vi "SiPM_Data_Analysis.vi"() -> ()   [LabVIEW 2019]
uses:
  <vilib>/Utility/error.llb/DialogType.ctl
  SiPM_Tests_Global_Var.vi
  Data_Analysis_subvis/ESA_Data_Analysis_Global_VIs.vi
  <vilib>/Analysis/NI_AALPro.lvlib
panel:
  out "property names":string[](array[string])
  out "property values":variant[](array[variant])
  out "data":waveform(dbl)[](array[waveform])
  out "Indicator":bool
  in  "Close Session":bool
  in  "Spectrum Calculation":bool=TRUE
  in  "Waveform Nb":u16
  in  "NbSamples":i64=100000 caption="Nb of Samples to Analyze" format="%.0p"
  in  "Refresh":bool
  in  "Load file to display":bool
  in  "Detailed":bool
  in  "Listbox":i32[](listbox) caption="Proton-Neutron_Brd.tdms"
  in  "Tab Control":enum32{"Waveform", "Calibration"}(tab)
  out "SiPM Waveform":waveform(dbl)[](graph)
  in  "X-Scale":bool
  in  "Calibrate":bool
  out "Offset":dbl step=0.001 format="%#_6p"
  out "Gain":dbl step=0.001 format="%#_6p"
  in  "Y2 (keV)":dbl
  in  "Y1 (keV)":dbl
  in  "AutoScale 4":bool
  out "Waveform Graph":dbl[][](graph)
  in  "Lower Cut-Off":dbl=50.0
  in  "Y-Scale 2":bool caption="Y-Scale"
  in  "CH1 Trigger Logic":T1(ring)=enum."Don't Care"
  in  "CH1 Trigger Thr":dbl=0.003 caption="CH1 Trigger Thr (V)" step=0.001 format="%#_6p"
  in  "Y-Scale":bool
  out "Nb of Selected Events":dbl step=0.001 format="%#_6p"
  out "Total Nb of Recorded Events":dbl step=0.001 format="%#_6p"
  in  "CH4 Trigger Logic":T1(ring)
  in  "CH4 Trigger Thr":dbl=0.003 caption="CH4 Trigger Thr (V)" step=0.001 format="%#_6p"
  in  "CH3 Trigger Logic":T1(ring)
  in  "CH3 Trigger":dbl=0.003 caption="CH3 Trigger Thr (V)" step=0.001 format="%#_6p"
  in  "CH2 Trigger Logic":T1(ring)=enum."Don't Care"
  in  "CH2 Trigger Thr":dbl=0.003 caption="CH2 Trigger Thr (V)" step=0.001 format="%#_6p"
  in  "AutoScale 3":bool
  in  "Update Energy":bool
  out "Energy_Spectr":T2(graph) caption="Spectrum"
  in  "Filter \nON?":bool
  in  "Threshold 2":dbl caption="Max_Value (V)" step=0.001 format="%#_6p"
  in  "Threshold":dbl caption="Energy Threshold (V)" step=0.001 format="%#_6p"
  out "Table":string[][](table)
  in  "Bin Min (V)":dbl=-0.0042 step=0.001 format="%#_6p"
  in  "Bin Max (V)":dbl=0.03005 step=0.001 format="%#_6p"
  out "Nb of Channels in Group":i32
  out "group names":string[](array[string])
  out "tdms file out":refnum<k34>
  in  "File contents":string[](tree)
  # "NCSR  DEMOKRITOS\nInstitute of Nuclear and Particle Physics\nDetectors Instrumentation Laboratory"
  # "SiPM Data Analysis"
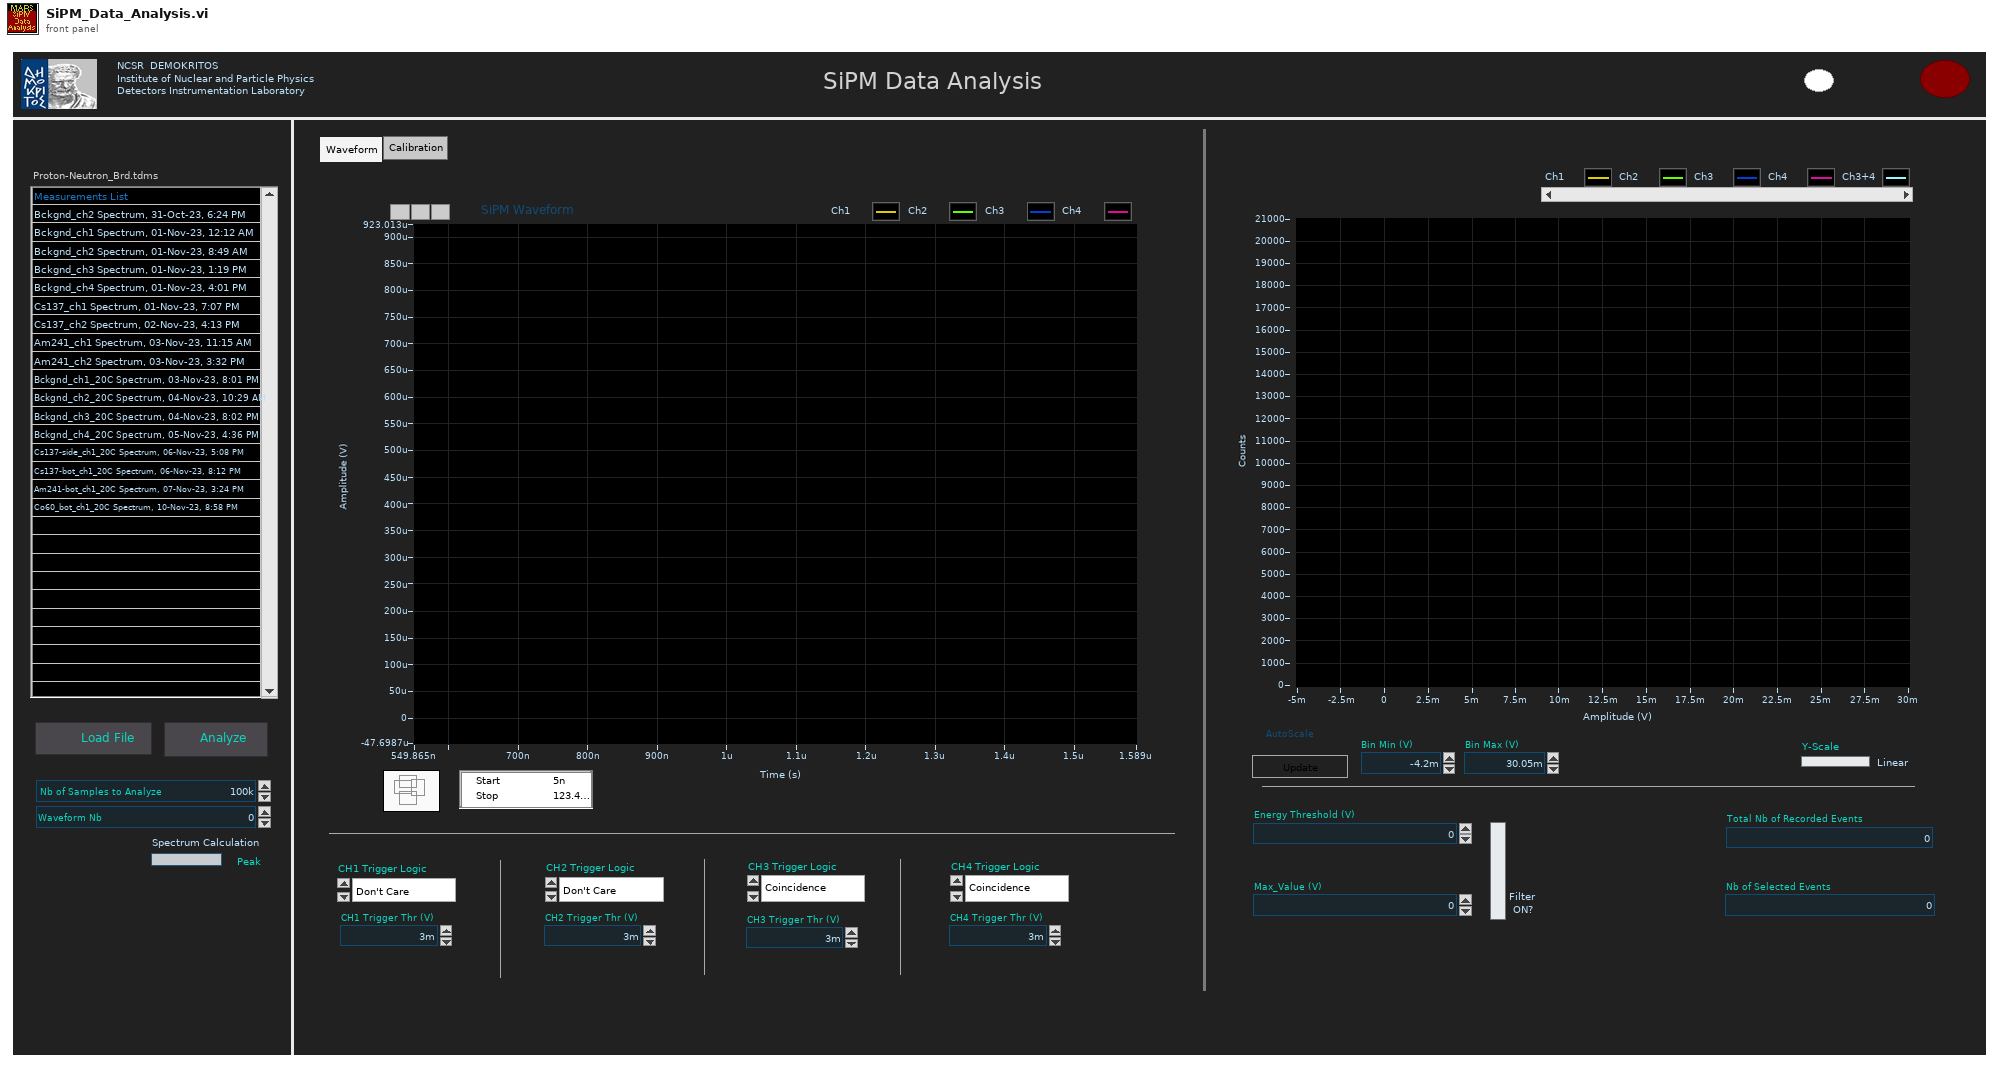
[diagram p1: front panel]
types:
  T1 = enum16{"Coincidence", "Anti-Coincidence", "Don't Care"}
  T2 = cluster{"X Values":dbl[], "Histogram: h(x)":i32[]}[]
  T3 = typedef "DialogType.ctl" = u16
  T4 = enum16{"open", "open or create", "create or replace", "create", "open (read-only)"}
  T5 = cluster{"X Values":dbl[], "Histogram: h(x)":i32[]}
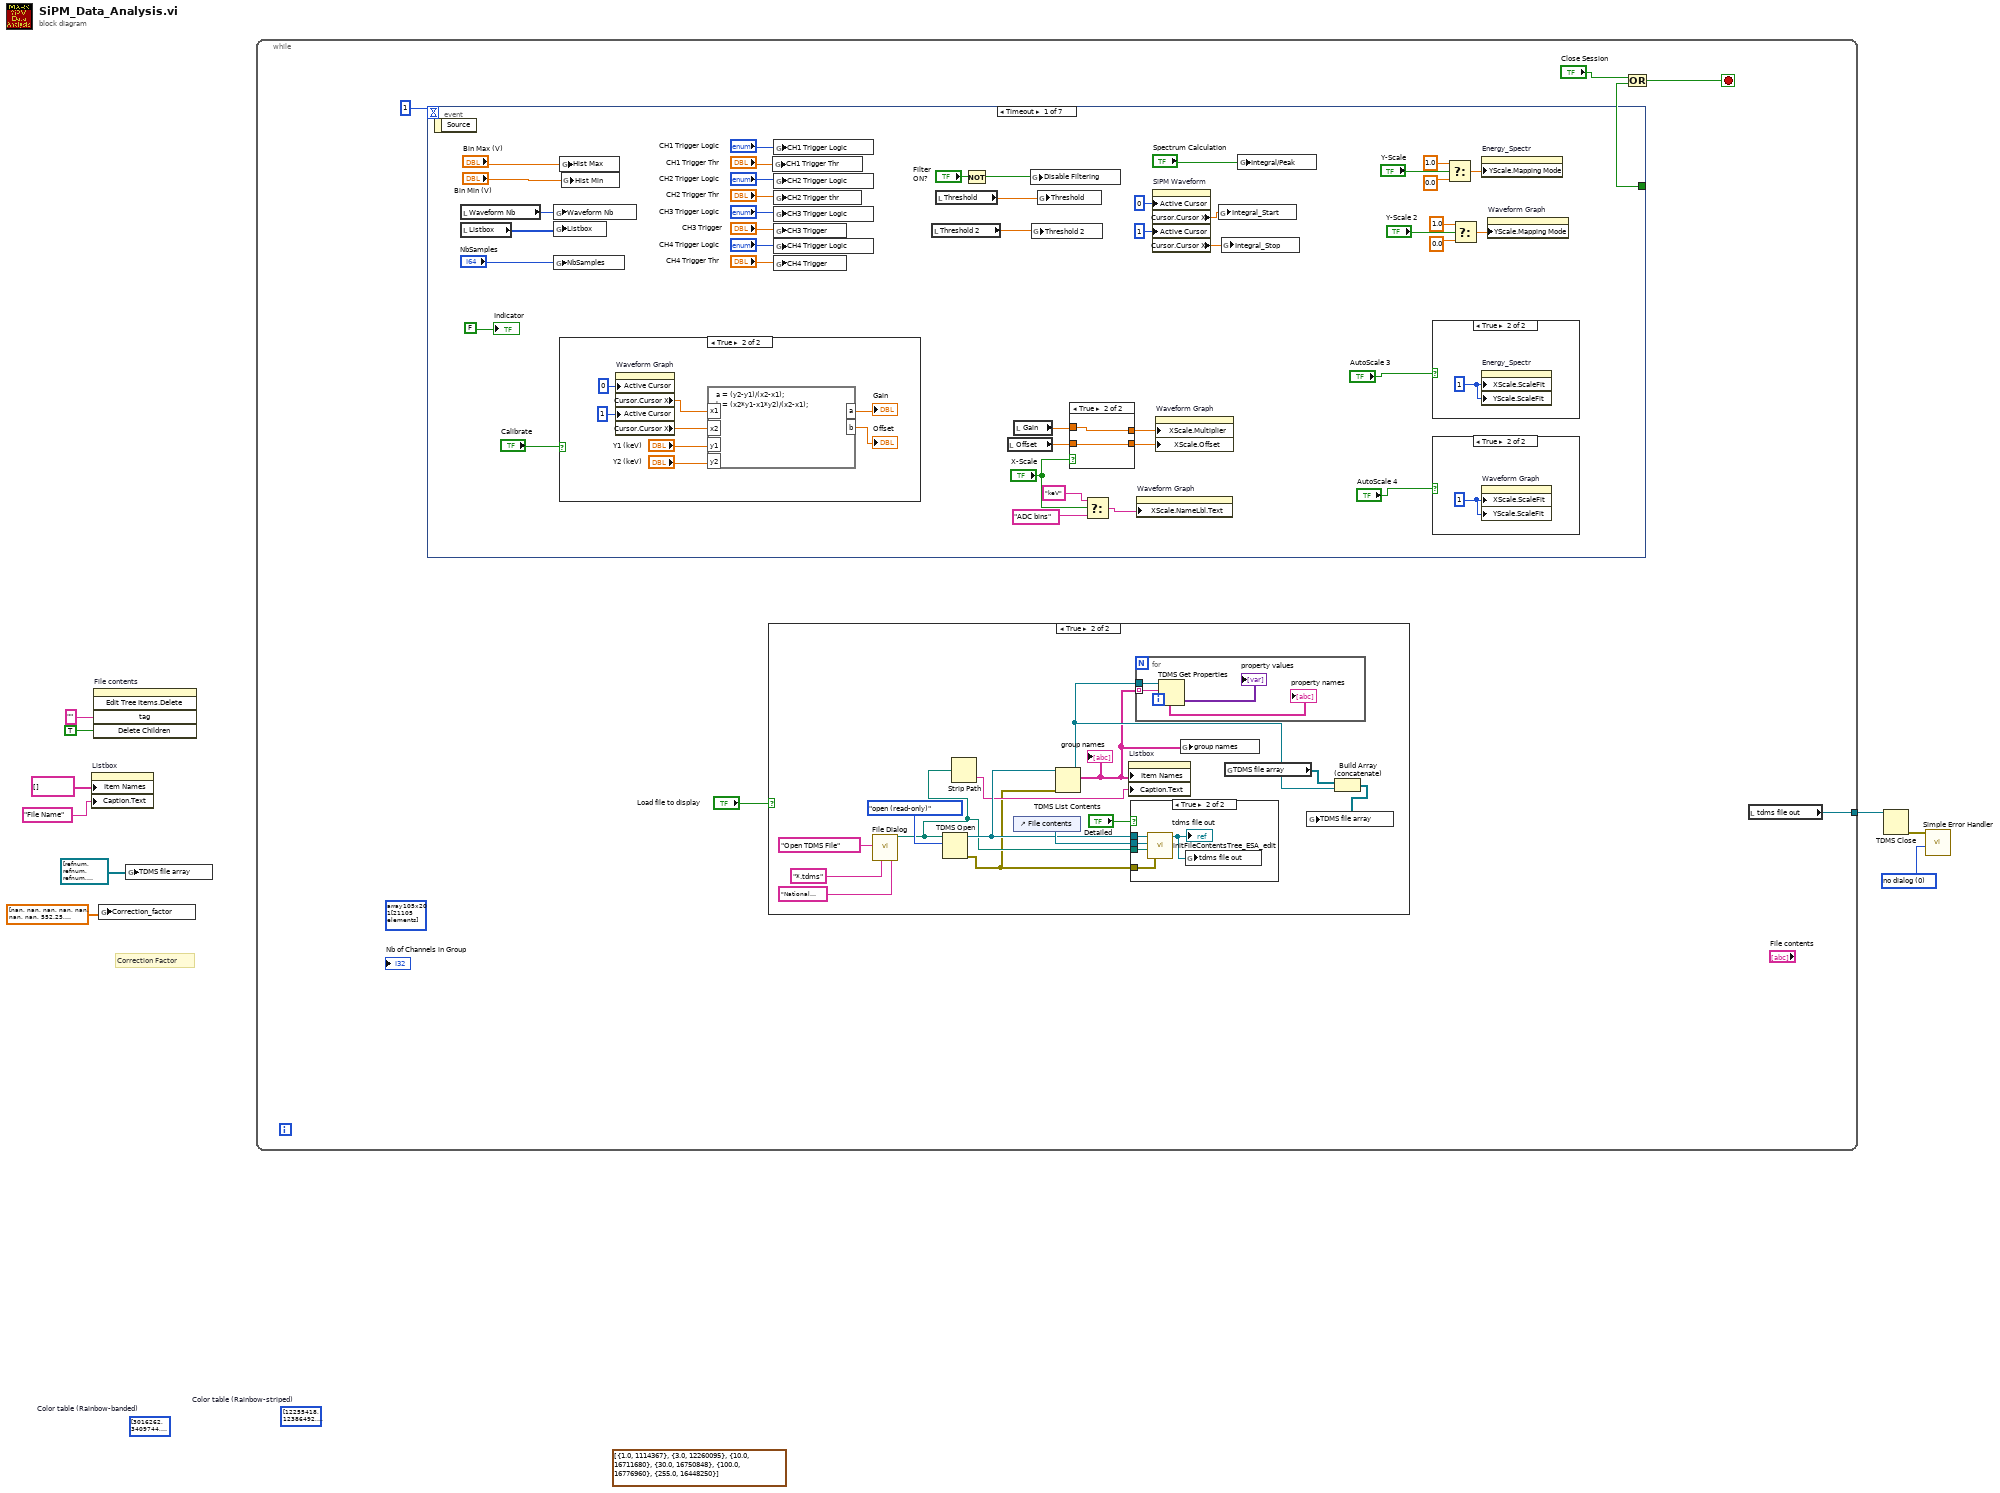
[diagram p0: block diagram]
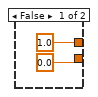
[diagram p2: hidden frame]
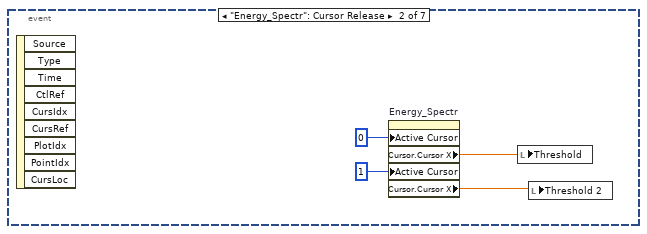
[diagram p6: hidden frame]
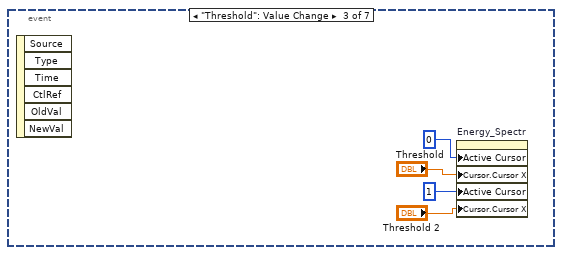
[diagram p7: hidden frame]
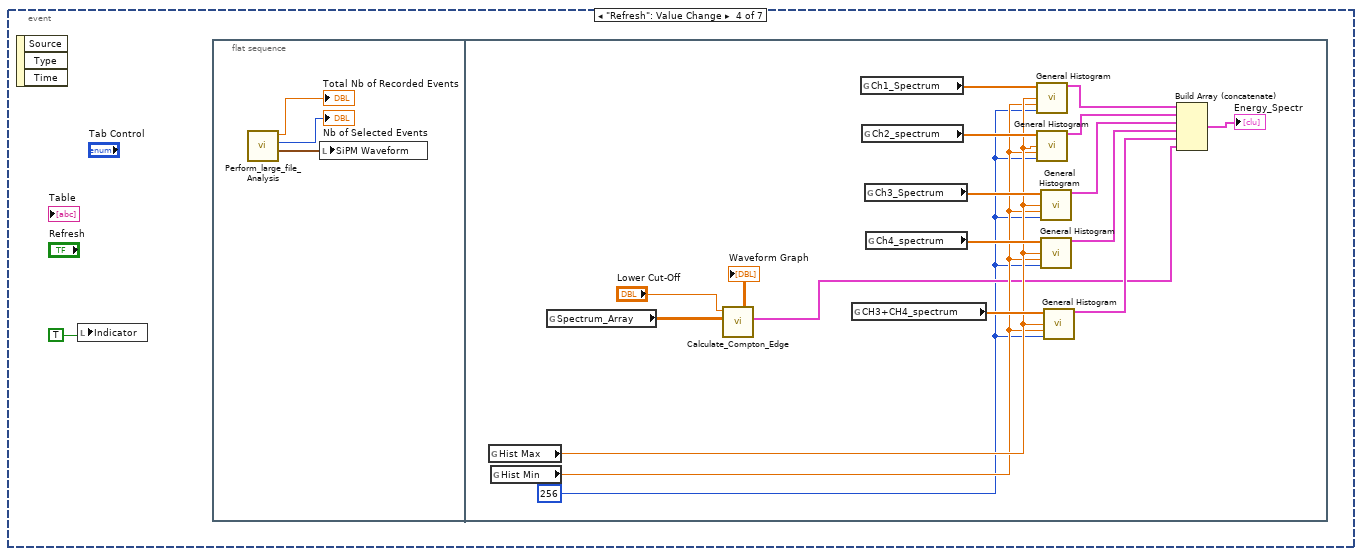
[diagram p8: hidden frame]
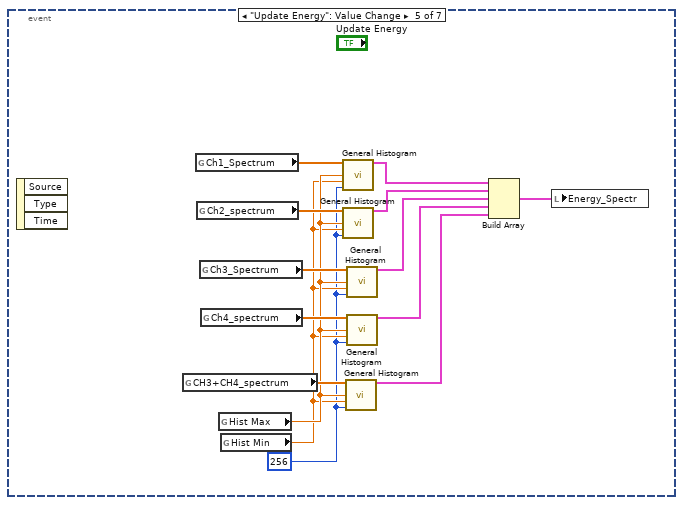
[diagram p9: hidden frame]
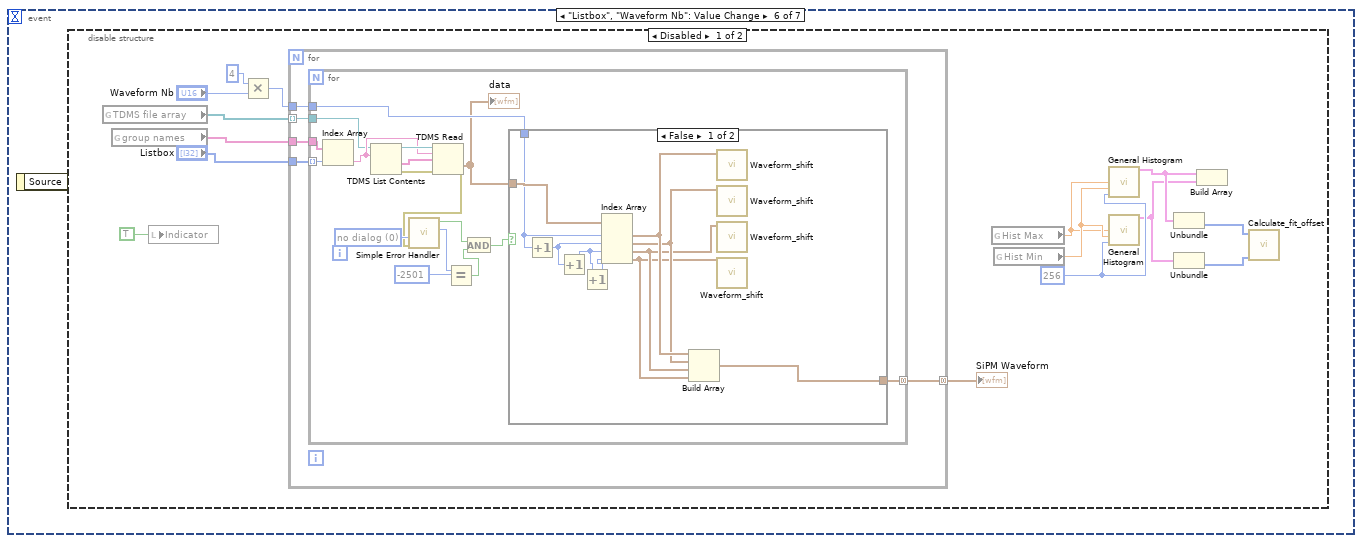
[diagram p10: hidden frame]
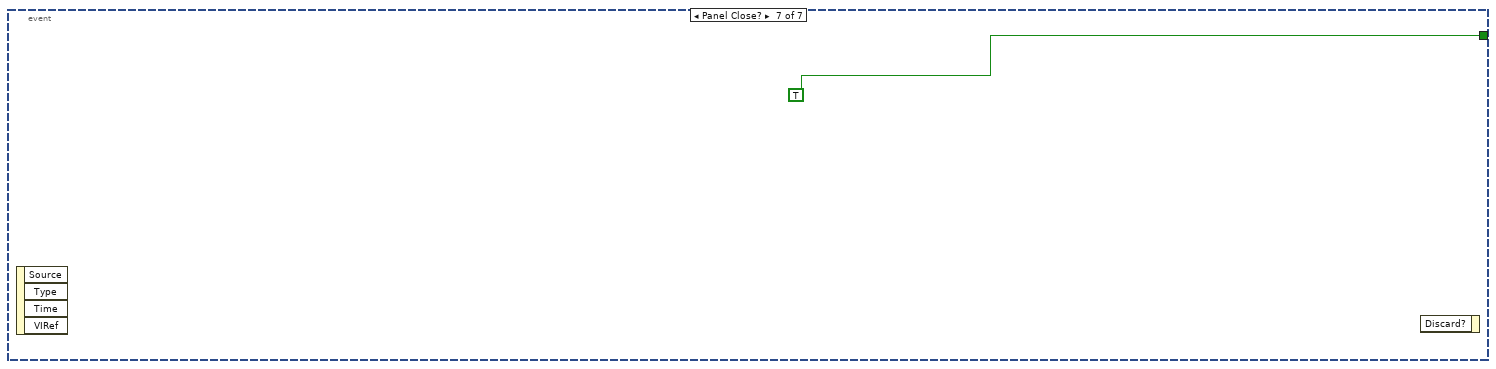
[diagram p13: hidden frame]
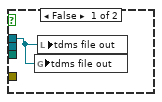
[diagram p15: hidden frame]
diagram:
  w2 = T3 0 items=["no dialog", "OK message", "continue or stop message", "OK message + warnings", "continue/stop + warnings"] ("type of dialog (OK msg:1)")
  (unwired) cluster{dbl, u32}[] [{1.0, 1114367}, {3.0, 12260095}, {10.0, 16711680}, {30.0, 16750848}, {100.0, 16776960}, {255.0, 16448250}] ("Z Scale.Marker Values[]")
  (unwired) u32[] [12255418, 12386492, 12517567, 12320960, 12189888, 12058817, 11927746, 11731139, 11600067, 9175197, 9044125, 11141318, 11010246, 10813639, 10682568, 10551497, 10354890, 10223818, 10092747, 7930019, 7798948, 9633997, 9502926, 9306319, 9175248, 9044176, 8847569, 8716498, 8585427, 6750377, 6619306, 8126677, 7995606, 7798999, 7667927, 7536856, 7340249, 7209178, 7078106, 5505199, 5374128, 6619357, 6488285, 6291678, 6160607, 6029536, 5832929, 5701857, 5570786, 4325557, 4194486, 5112036, 4980965, 4784358, 4653287, 4522215, 4325608, 4194537, 4063466, 3080380, 3014844, 3604716, 3408109, 3277038, 3277038, 3145966, 3014895, 2818288, 2687217, 2556145, 1900738, 1769666, 2097396, 1900789, 1769717, 1638646, 1507575, 1310968, 1179896, 1048825, 721096, 590024, 590075, 393468, 262397, 131326, 255, 1791, 3327, 4863, 5068, 6348, 9471, 11007, 12543, 14079, 15615, 17151, 18687, 20223, 17612, 18636, 25087, 26623, 28159, 29695, 31231, 32767, 34303, 35839, 29900, 31180, 40447, 41983, 43775, 45311, 46847, 48383, 49919, 51455, 42444, 43724, 56063, 57599, 59135, 60671, 62207, 63743, 65535, 65528, 52418, 52413, 65510, 65504, 65498, 65492, 65486, 65480, 65474, 65468, 52369, 52364, 65449, 65443, 65437, 65431, 65425, 65419, 65413, 65407, 52321, 52316, 65389, 65383, 65377, 65371, 65364, 65358, 65352, 65346, 52272, 52267, 65328, 65322, 65316, 65310, 65304, 65298, 65292, 65286, 52224, 314368, 851712, 1244928, 1638144, 2031360, 2424576, 2817792, 3211008, 3604224, 3197952, 3525632, 4783872, 5177088, 5635840, 6029056, 6422272, 6815488, 7208704, 7601920, 6409216, 6736896, 6736896, 8781568, 9174784, 9568000, 9961216, 10354432, 10747648, 11206400, 11599616, 9554944, 9882624, 12779264, 13172480, 13565696, 13958912, 14352128, 14745344, 15138560, 15531776, 12766208, 13093888, 16776960, 16775170, 16773637, 16771847, 16770314, 16768780, 16766991, 16765457, 13411088, 13409810, 16760601, 16758812, 16757278, 16755745, 16753955, 16752422, 16750888, 16749099, 13398052, 13396774, 16744243, 16742704, 16741166, 16739884, 16738345, 16736807, 16735269, 16733730, 13385753, 13384728, 16729371, 16727833, 16726295, 16725012, 16723474, 16721936, 16720397, 16718859, 13373959, 13372677, 16714500, 16712962, 16711680]  # Color table (Rainbow-striped)
  (unwired) u32[] [3016262, 3409744, 4000097, 4721526, 5508493, 6229924, 6820281, 7214025, 7345364, 7279831, 6886611, 6362057, 5640632, 4788132, 4001165, 3214197, 2492769, 2033488, 1640006, 1508930, 1508934, 1640272, 1902945, 2165622, 2428301, 2690980, 2822585, 2888649, 2757844, 2626775, 2299091, 1971145, 1642936, 1249188, 920973, 724086, 592737, 461392, 395846, 396098, 396358, 462928, 595297, 727925, 861069, 994212, 1127608, 1260745, 1328083, 1329111, 1329876, 1264073, 1132217, 999844, 866957, 734070, 600929, 468304, 401734, 401730, 402502, 469584, 603489, 737909, 737909, 872845, 1008036, 1143224, 1277641, 1345747, 1347287, 1347796, 1281225, 1147833, 1013668, 878989, 743798, 609121, 475216, 407878, 407362, 408390, 476496, 611681, 747893, 884877, 1022116, 1158840, 1294793, 1363667, 1365719, 1365202, 1296836, 1161649, 1025178, 888194, 751211, 614742, 479302, 411196, 410168, 411193, 479297, 614732, 750939, 888171, 1025145, 1161350, 1296782, 1364883, 1365906, 1365132, 1296769, 1161588, 1025124, 888147, 751172, 614710, 479276, 411173, 410146, 411170, 479270, 614700, 750900, 888124, 1025091, 1161289, 1296716, 1364813, 1365834, 1365062, 1296703, 1161527, 1025070, 888101, 751133, 614678, 479249, 411149, 410124, 411147, 479244, 614668, 750861, 888078, 1156111, 1488913, 1820947, 2151188, 2414356, 2610196, 2738451, 2668817, 2597903, 2329869, 2061835, 1794313, 1593351, 1459718, 1458694, 1590790, 1921031, 2449673, 3110155, 3902733, 4695055, 5486609, 6211859, 6738708, 7132948, 7197716, 7063827, 6666513, 6136847, 5410061, 4617739, 3957001, 3362823, 2967046, 2900486, 3098118, 3690503, 4546825, 5666059, 6917389, 8233999, 9484305, 10537235, 11326228, 11786004, 11785236, 11785236, 11454739, 10729745, 9675791, 8424717, 7173643, 6054153, 5066759, 4474374, 4342278, 4605190, 5262855, 6380553, 7695883, 9273613, 10785807, 12100625, 13217555, 13874452, 14136340, 13938196, 13214227, 12161553, 10780431, 9267725, 7755531, 6374921, 5257479, 4599814, 4336646, 4599302, 5255943, 6372361, 7685899, 9261837, 10771983, 12085009, 13200659, 13856532, 14118164, 13920276, 13197075, 12145937, 10766351, 9255949, 7745547, 6366729, 5250567, 4593926, 4331014, 4593158, 5249287, 6364169, 7675915, 9249805, 10758159, 12069393, 13183507, 13838612, 14099988, 13902356, 13180179, 12130065, 10752527]  # Color table (Rainbow-banded)
  # "Correction Factor"
  n1 = property on="Listbox" class="LstBox (strict)"("Item Names"=string[] [], "Caption.Text"="File Name") -> ()  [unwired: 2 in, 2 out]
  n2 = invoke on="File contents" class="Tree (strict)" method="Edit Tree Items.Delete"("tag"="" ("Tag"), "Delete Children"=TRUE ("Delete Children?")) -> ()  [unwired: 3 in, 5 out]
  n3 = global write "SiPM_Tests_Global_Var.vi" "Correction_factor"(dbl[] [nan, nan, nan, nan, nan, nan, nan, 552.25, 547.2727272727273, 556.8888888888889, 571.6521739130435, 581.5526315789474, 593.6590909090909, 606.7333333333333, 610.4848484848485, 619.9565217391304, 624.8125, 628.375, 631.8064516129032, 637.0434782608696, 640.92, 643.5, 643.92, 647.7619047619048, 650.1923076923077, 651.5714285714286, 652.375, 654.9130434782609, 656.35, 658.4117647058823, 658.5909090909091, 660.0952380952381, 662.3157894736842, 661.5, 663.4166666666666, 665.8888888888889, 666.0, 666.0, 667.8421052631579, 668.2727272727273, 669.7, 671.4166666666666, 671.2631578947369, 672.2272727272727, 672.0588235294117, 674.0952380952381, 673.0, 674.0526315789474, 675.6111111111111, 677.1578947368421, 677.9411764705883, 676.5263157894736, 677.0666666666667, 678.0, 677.3333333333334, 678.8333333333334, 678.4, 680.0, 680.0666666666667, 680.625, 678.8823529411765, 681.1764705882352, 680.3333333333334, 681.1052631578947, 681.4375, 683.1052631578947, 682.6875, 682.7222222222222, 683.4666666666667, 684.1052631578947, 682.8461538461538, 685.375, 684.5, 684.8333333333334, 683.8, 684.6111111111111, 685.7142857142857, 686.5555555555555, 684.2857142857143, 685.4444444444445, 685.4375, 686.0, 686.375, 687.1176470588235, 685.3125, 685.9333333333333, 687.0, 686.0, 686.1538461538462, 686.75, 686.7272727272727, 686.875, 687.4444444444445, 686.5, 686.3076923076923, 685.8461538461538, 688.3, 688.3571428571429, 685.8571428571429, 688.4166666666666, 687.4, 687.8, 687.1818181818181, 687.9230769230769, 687.5, 688.7857142857143, 685.5714285714286, 686.9090909090909, 688.2, 690.5555555555555, 688.5, 689.6923076923077, 689.6, 690.1111111111111, 692.5, 687.6666666666666, 688.0, 686.0, 690.5, 690.0, 688.6666666666666, nan, 691.75, 682.0, 687.5, 692.5, 690.0, 687.0, 686.3333333333334, 693.5, 689.5, 689.5, nan, nan, 693.0, nan, 686.0, nan, nan, nan, 690.0, 690.0, nan, nan, nan, nan, nan, nan, nan, nan, nan, nan, nan, nan, nan, nan, nan, nan, nan, nan, nan, nan, nan, nan, nan, nan, nan, nan, nan, nan, nan, nan, nan, nan, nan, nan, nan, nan, nan, nan, nan, nan, nan, nan, nan, nan, nan, nan, nan, nan, nan, nan, nan, nan, nan, nan, nan, nan, nan, nan, nan, nan, nan, nan, nan, nan, nan, nan, nan, nan, nan, nan, nan, nan, nan, nan, nan, nan, nan, nan, nan, nan, nan, nan, nan, nan, nan, nan, nan, nan, nan, nan, nan, nan, nan, nan, nan, nan, nan, nan, nan, nan, nan, nan, nan, nan, nan, nan, nan, nan, nan, nan, nan, nan, nan, nan, nan] ("Correction_factor")) -> ()
  n4 = global write "SiPM_Tests_Global_Var.vi" "TDMS file array"(refnum<k34>[] [refnum, refnum, refnum, refnum] ("TDMS file array")) -> ()
  n5 = while {
    tunnel: [w14] -> w9
    stop <- w13 stop-if-true
    (unwired) i32[][] array105x201[21105 elements] ("spectrum")
    n6 = event shown="[0] Timeout" {
      selector: _ -> [_ _ _ _ _ _ _]
      dyn-events: _ -> [_ _ _ _ _ _ _]
      timeout: 1 -> [_ _ _ _ _ _ _]
      tunnel: [_ _ _ _ _ _ TRUE ("Stop Button")] -> w12
      event Timeout {
        n7 = event-data() -> ()  [unwired: 1 in, 1 out]
        n8 = local read "Waveform Nb"() -> (w51:u16)
        n9 = local read "Listbox"() -> (w54:i32[])
        n10 = global write "SiPM_Tests_Global_Var.vi" "Waveform Nb"(w51) -> ()
        n11 = global write "ESA_Data_Analysis_Global_VIs.vi" "Listbox"(w54) -> ()
        n12 = global write "SiPM_Tests_Global_Var.vi" "NbSamples"("NbSamples") -> ()
        n13 = global write "SiPM_Tests_Global_Var.vi" "Hist Max"("Bin Max (V)") -> ()
        n14 = case shown="True" "Calibrate" {
          frame False {
          }
          frame True {
            n15 = property on="Waveform Graph" class="WFGraph (strict)"("Active Cursor"=u32 0, "Active Cursor"=u32 1) -> ("Cursor.Cursor X"=w67:dbl, "Cursor.Cursor X"=w66:dbl)  [unwired: 2 in, 2 out]
            n16 = formula code="a = (y2-y1)/(x2-x1);\nb = (x2*y1-x1*y2)/(x2-x1);"("x1"=w67, "x2"=w66, "y1"="Y1 (keV)", "y2"="Y2 (keV)") -> ("a"=→"Gain":dbl, "b"=→"Offset":dbl)
          }
        }
        n17 = global write "SiPM_Tests_Global_Var.vi" "Hist Min"("Bin Min (V)") -> ()
        n18 = global write "SiPM_Tests_Global_Var.vi" "CH1 Trigger Thr"("CH1 Trigger Thr") -> ()
        n19 = global write "SiPM_Tests_Global_Var.vi" "CH1 Trigger Logic"("CH1 Trigger Logic") -> ()
        n20 = global write "SiPM_Tests_Global_Var.vi" "CH2 Trigger Logic"("CH2 Trigger Logic") -> ()
        n21 = global write "SiPM_Tests_Global_Var.vi" "CH2 Trigger thr"("CH2 Trigger Thr") -> ()
        n22 = global write "SiPM_Tests_Global_Var.vi" "CH3 Trigger Logic"("CH3 Trigger Logic") -> ()
        n23 = global write "SiPM_Tests_Global_Var.vi" "CH3 Trigger"("CH3 Trigger") -> ()
        n24 = global write "SiPM_Tests_Global_Var.vi" "CH4 Trigger Logic"("CH4 Trigger Logic") -> ()
        n25 = global write "SiPM_Tests_Global_Var.vi" "CH4 Trigger"("CH4 Trigger Thr") -> ()
        n26 = local read "Threshold 2"() -> (w50:dbl)
        n27 = local read "Threshold"() -> (w52:dbl)
        n28 = Not(x="Filter \nON?") -> (.not. x?=w48:bool)
        n29 = local read "Offset"() -> (w20:dbl)
        n30 = local read "Gain"() -> (w21:dbl)
        n31 = global write "SiPM_Tests_Global_Var.vi" "Disable Filtering"(w48) -> ()
        n32 = global write "SiPM_Tests_Global_Var.vi" "Threshold 2"(w50) -> ()
        n33 = global write "SiPM_Tests_Global_Var.vi" "Threshold"(w52) -> ()
        n34 = case shown="True" "X-Scale" {
          tunnel: [1.0 ("gain") w61] -> w23
          tunnel: w21 -> [_ w61]
          tunnel: [0.0 ("offset") w60] -> w22
          tunnel: w20 -> [_ w60]
          frame False {
          }
          frame True {
          }
        }
        n35 = Select(t="keV" ("X Scale.Unit Label.Text"), s="X-Scale", f="ADC bins" ("X Scale.Unit Label.Text")) -> (s? t:f=w16:string)
        n36 = property on="Waveform Graph" class="WFGraph (strict)"("XScale.NameLbl.Text"=w16) -> ()  [unwired: 2 in, 2 out]
        n37 = property on="SiPM Waveform" class="WFGraph (strict)"("Active Cursor"=u32 0, "Active Cursor"=u32 1) -> ("Cursor.Cursor X"=w45:dbl, "Cursor.Cursor X"=w44:dbl)  [unwired: 2 in, 2 out]
        n38 = property on="Waveform Graph" class="WFGraph (strict)"("XScale.Multiplier"=w23, "XScale.Offset"=w22) -> ()  [unwired: 2 in, 2 out]
        n39 = global write "SiPM_Tests_Global_Var.vi" "Integral_Start"(w45) -> ()
        n40 = global write "SiPM_Tests_Global_Var.vi" "Integral_Stop"(w44) -> ()
        n41 = global write "SiPM_Tests_Global_Var.vi" "Integral/Peak"("Spectrum Calculation") -> ()
        n42 = case shown="True" "AutoScale 3" {
          frame False {
          }
          frame True {
            w70 = u8 1 ("X Scale.Scale Fit")
            n43 = property on="Energy_Spectr" class="XYGraph (strict)"("XScale.ScaleFit"=w70, "YScale.ScaleFit"=w70) -> ()  [unwired: 2 in, 2 out]
          }
        }
        n44 = case shown="True" "AutoScale 4" {
          frame False {
          }
          frame True {
            w71 = u8 1 ("X Scale.Scale Fit")
            n45 = property on="Waveform Graph" class="WFGraph (strict)"("XScale.ScaleFit"=w71, "YScale.ScaleFit"=w71) -> ()  [unwired: 2 in, 2 out]
          }
        }
        n46 = Select(t=1.0, s="Y-Scale", f=0.0 ("t")) -> (s? t:f=w36:dbl)
        n47 = Select(t=1.0, s="Y-Scale 2", f=0.0 ("t")) -> (s? t:f=w28:dbl)
        n48 = property on="Energy_Spectr" class="XYGraph (strict)"("YScale.Mapping Mode"=w36) -> ()  [unwired: 2 in, 2 out]
        n49 = property on="Waveform Graph" class="WFGraph (strict)"("YScale.Mapping Mode"=w28) -> ()  [unwired: 2 in, 2 out]
        "Indicator" <- FALSE ("Indicator")
      }
      event "Energy_Spectr": Cursor Release {
        n50 = event-data() -> ()  [unwired: 1 in, 9 out]
        n51 = property on="Energy_Spectr" class="XYGraph (strict)"("Active Cursor"=u32 0, "Active Cursor"=u32 1) -> ("Cursor.Cursor X"=w75:dbl, "Cursor.Cursor X"=w72:dbl)  [unwired: 2 in, 2 out]
        n52 = local write "Threshold"(w75) -> ()
        n53 = local write "Threshold 2"(w72) -> ()
      }
      event "Threshold": Value Change {
        n54 = event-data() -> ()  [unwired: 1 in, 6 out]
        n55 = property on="Energy_Spectr" class="XYGraph (strict)"("Active Cursor"=u32 0, "Cursor.Cursor X"="Threshold", "Active Cursor"=u32 1, "Cursor.Cursor X"="Threshold 2") -> ()  [unwired: 2 in, 2 out]
      }
      event "Refresh": Value Change {
        n56 = event-data() -> ()  [unwired: 1 in, 3 out]
        n57 = local write "Indicator"(TRUE ("Indicator")) -> ()
        n58 = flat-sequence {
          frame #0 {
            n59 = call "Perform_large_file_Analysis.vi"() -> ("Wvfm"=w83:waveform(dbl)[], "Filtered Nb of Events"=→"Nb of Selected Events":i32, "Total Nb of Events"=→"Total Nb of Recorded Events":dbl)  [unwired: 6 in]
            n60 = local write "SiPM Waveform"(w83) -> ()
          }
          frame #1 {
            w84 = 256 ("# bins")
            n61 = global read "SiPM_Tests_Global_Var.vi" "Hist Max"() -> (w89:dbl)
            n62 = global read "SiPM_Tests_Global_Var.vi" "Hist Min"() -> (w88:dbl)
            n63 = global read "SiPM_Tests_Global_Var.vi" "Spectrum_Array"() -> (w90:dbl[][])
            n64 = call "Calculate_Compton_Edge.vi"("Spectrum_Array"=w90, "Lower Cut-Off"="Lower Cut-Off") -> ("Array"=w87:T2, "Waveform Graph"=→"Waveform Graph":dbl[][])  [unwired: 8 in]
            n65 = global read "SiPM_Tests_Global_Var.vi" "CH3+CH4_spectrum"() -> (w92:dbl[])
            n66 = global read "SiPM_Tests_Global_Var.vi" "Ch1_Spectrum"() -> (w100:dbl[])
            n67 = global read "SiPM_Tests_Global_Var.vi" "Ch2_spectrum"() -> (w101:dbl[])
            n68 = global read "SiPM_Tests_Global_Var.vi" "Ch3_Spectrum"() -> (w96:dbl[])
            n69 = global read "SiPM_Tests_Global_Var.vi" "Ch4_spectrum"() -> (w95:dbl[])
            n70 = call <vilib>:"General Histogram.vi"("X"=w100, "max"=w89, "min"=w88, "# bins"=w84) -> ("Histogram Graph"=w98:T5)  [unwired: 7 in, 4 out]
            n71 = call <vilib>:"General Histogram.vi"("X"=w101, "max"=w89, "min"=w88, "# bins"=w84) -> ("Histogram Graph"=w97:T5)  [unwired: 7 in, 4 out]
            n72 = call <vilib>:"General Histogram.vi"("X"=w96, "max"=w89, "min"=w88, "# bins"=w84) -> ("Histogram Graph"=w94:T5)  [unwired: 7 in, 4 out]
            n73 = call <vilib>:"General Histogram.vi"("X"=w95, "max"=w89, "min"=w88, "# bins"=w84) -> ("Histogram Graph"=w93:T5)  [unwired: 7 in, 4 out]
            n74 = call <vilib>:"General Histogram.vi"("X"=w92, "max"=w89, "min"=w88, "# bins"=w84) -> ("Histogram Graph"=w91:T5)  [unwired: 7 in, 4 out]
            n75 = Build Array (concatenate)(w98, w97, w94, w93, w91, w87) -> (→"Energy_Spectr":T2)
          }
        }
      }
      event "Update Energy": Value Change {
        w103 = 256 ("# bins")
        n76 = event-data() -> ()  [unwired: 1 in, 3 out]
        n77 = global read "SiPM_Tests_Global_Var.vi" "CH3+CH4_spectrum"() -> (w106:dbl[])
        n78 = global read "SiPM_Tests_Global_Var.vi" "Ch1_Spectrum"() -> (w114:dbl[])
        n79 = global read "SiPM_Tests_Global_Var.vi" "Ch2_spectrum"() -> (w115:dbl[])
        n80 = global read "SiPM_Tests_Global_Var.vi" "Ch3_Spectrum"() -> (w111:dbl[])
        n81 = global read "SiPM_Tests_Global_Var.vi" "Ch4_spectrum"() -> (w110:dbl[])
        n82 = global read "SiPM_Tests_Global_Var.vi" "Hist Max"() -> (w105:dbl)
        n83 = global read "SiPM_Tests_Global_Var.vi" "Hist Min"() -> (w104:dbl)
        n84 = call <vilib>:"General Histogram.vi"("X"=w114, "max"=w105, "min"=w104, "# bins"=w103) -> ("Histogram Graph"=w113:T5)  [unwired: 7 in, 4 out]
        n85 = call <vilib>:"General Histogram.vi"("X"=w115, "max"=w105, "min"=w104, "# bins"=w103) -> ("Histogram Graph"=w112:T5)  [unwired: 7 in, 4 out]
        n86 = call <vilib>:"General Histogram.vi"("X"=w106, "max"=w105, "min"=w104, "# bins"=w103) -> ("Histogram Graph"=w102:T5)  [unwired: 7 in, 4 out]
        n87 = call <vilib>:"General Histogram.vi"("X"=w111, "max"=w105, "min"=w104, "# bins"=w103) -> ("Histogram Graph"=w109:T5)  [unwired: 7 in, 4 out]
        n88 = call <vilib>:"General Histogram.vi"("X"=w110, "max"=w105, "min"=w104, "# bins"=w103) -> ("Histogram Graph"=w108:T5)  [unwired: 7 in, 4 out]
        n89 = Build Array(w113, w112, w109, w108, w102) -> (w107:T2)
        n90 = local write "Energy_Spectr"(w107) -> ()
      }
      event "Listbox", "Waveform Nb": Value Change {
        n91 = event-data() -> ()  [unwired: 1 in, 1 out]
        n92 = disable-structure shown="Disabled" {
          frame Disabled {
            w120 = 256 ("# bins")
            n93 = global read "SiPM_Tests_Global_Var.vi" "TDMS file array"() -> (w129:refnum<k34>[])
            n94 = global read "ESA_Data_Analysis_Global_VIs.vi" "group names"() -> (w130:string[])
            n95 = local write "Indicator"(TRUE ("Indicator")) -> ()
            n96 = Multiply(x=4, y="Waveform Nb") -> (x*y=w125:i32)
            n97 = for {
              tunnel: "Listbox" -> [w135]
              tunnel: w130 -> [w134]
              tunnel: w129 -> [w133] mode=indexing
              tunnel: [w132] -> w123 mode=concatenating
              tunnel: w125 -> [w131]
              n98 = for {
                tunnel: w135 -> [w148] mode=indexing
                tunnel: w134 -> [w147]
                tunnel: w133 -> [w146]
                tunnel: [w145] -> w132 mode=concatenating
                tunnel: w131 -> [w137]
                w144 = T3 0 items=["no dialog", "OK message", "continue or stop message", "OK message + warnings", "continue/stop + warnings"] ("type of dialog (OK msg:1)")
                n99 = Index Array(array=w147, index=w148) -> (element=w151:string)
                n100 = TDMS List Contents(6:w151, 7:w146) -> (0:w149:errorcluster, 1:w150:string[], 3:w152:refnum<k34>)  [unwired: 1 in, 1 out]
                n101 = TDMS Read(0:w152, 5:w151, 7:w150, 11:w149) -> (10:w136:waveform(dbl)[], 15:w140:errorcluster)  [unwired: 4 in, 4 out]
                "data" <- w136
                n102 = call <vilib>:"Simple Error Handler.vi"("type of dialog (OK msg:1)"=w144, "error in (no error)"=w140) -> ("error?"=w139:bool, "code out"=w143:i32)  [unwired: 3 in, 3 out]
                n103 = Equal?(x=w143, y=-2501) -> (x = y?=w141:bool)
                n104 = And(x=w139, y=w141) -> (x .and. y?=w138:bool)
                n105 = case shown="False" w138 {
                  tunnel: w136 -> [w162 _]
                  tunnel: [w158 _] -> w145
                  tunnel: w137 -> [w161 _]
                  frame False {
                    n106 = Increment(x=w161) -> (x+1=w157:i32)
                    n107 = Increment(x=w157) -> (x+1=w155:i32)
                    n108 = Increment(x=w155) -> (x+1=w156:i32)
                    n109 = Index Array(array=w162, index #1=w161, index #2=w157, index #3=w155, index #4=w156) -> (element #1=w160:waveform(dbl), element #2=w159:waveform(dbl), element #3=w154:waveform(dbl), element #4=w153:waveform(dbl))
                    n110 = Build Array(w160, w159, w154, w153) -> (w158:waveform(dbl)[])
                    n111 = call "Waveform_shift.vi"("Waveform_in"=w160) -> ()  [unwired: 9 in, 1 out]
                    n112 = call "Waveform_shift.vi"("Waveform_in"=w159) -> ()  [unwired: 9 in, 1 out]
                    n113 = call "Waveform_shift.vi"("Waveform_in"=w154) -> ()  [unwired: 9 in, 1 out]
                    n114 = call "Waveform_shift.vi"("Waveform_in"=w153) -> ()  [unwired: 9 in, 1 out]
                  }
                  frame True {
                  }
                }
              }
            }
            "SiPM Waveform" <- w123
            n115 = global read "SiPM_Tests_Global_Var.vi" "Hist Max"() -> (w121:dbl)
            n116 = global read "SiPM_Tests_Global_Var.vi" "Hist Min"() -> (w122:dbl)
            n117 = call <vilib>:"General Histogram.vi"("max"=w121, "min"=w122, "# bins"=w120) -> ("Histogram Graph"=w119:T5)  [unwired: 8 in, 4 out]
            n118 = call <vilib>:"General Histogram.vi"("max"=w121, "min"=w122, "# bins"=w120) -> ("Histogram Graph"=w118:T5)  [unwired: 8 in, 4 out]
            n119 = Unbundle(w119) -> ("Histogram: h(x)"=w117:i32[])  [unwired: 1 out]
            n120 = Unbundle(w118) -> ("Histogram: h(x)"=w116:i32[])  [unwired: 1 out]
            n121 = Build Array(w119, w118) -> ()  [unwired: 1 out]
            n122 = call "Calculate_fit_offset.vi"("baseline1"=w117, "baseline2"=w116) -> ()  [unwired: 4 in, 4 out]
          }
          frame Enabled {
          }
        }
      }
      event Panel Close? {
        n123 = event-data() -> ()  [unwired: 1 in, 4 out]
        n124 = event-data() -> ()  [unwired: 2 in, 1 out]
      }
    }
    n125 = case shown="True" "Load file to display" {
      frame False {
      }
      frame True {
        n126 = call "File Dialog"("prompt"="Open TDMS File" ("prompt tdms"), "pattern (all files)"="*.tdms", "pattern label"="National Instruments TDM Streaming" ("pattern label tdms")) -> ("selected path"=w171:path)  [unwired: 4 in, 8 out]
        n127 = TDMS Open(10:T4."open (read-only)" ("operation (0:open)"), 11:w171) -> (0:w168:errorcluster, 3:w172:refnum<k34>)  [unwired: 5 in]
        n128 = Strip Path(path=w171) -> (name=w170:string)  [unwired: 1 out]
        n129 = control-ref of="File contents"() -> (w177:refnum<vi>)
        n130 = TDMS List Contents(4:w168, 7:w172) -> (2:w164:string[], 3:w165:refnum<k34>)  [unwired: 1 in, 2 out]
        "group names" <- w164
        n131 = property on="Listbox" class="LstBox (strict)"("Item Names"=w164, "Caption.Text"=w170) -> ()  [unwired: 2 in, 2 out]
        n132 = case shown="True" "Detailed" {
          tunnel: w177 -> [_ w187]
          tunnel: w168 -> [_ w186]
          tunnel: w171 -> [_ w185]
          tunnel: w172 -> [w182 w184]
          frame False {
            n133 = global write "ESA_Data_Analysis_Global_VIs.vi" "tdms file out"(w182) -> ()
            n134 = local write "tdms file out"(w182) -> ()
          }
          frame True {
            n135 = call "initFileContentsTree_ESA_edit.vi"("error in (no error)"=w186, "file path"=w185, "Tree Refnum"=w187, "tdms file"=w184) -> ("tdms file out"=w183:refnum<k34>)  [unwired: 2 in, 1 out]
            "tdms file out" <- w183
            n136 = global write "ESA_Data_Analysis_Global_VIs.vi" "tdms file out"(w183) -> ()
          }
        }
        n137 = for {
          tunnel: w165 -> [w181]
          tunnel: w164 -> [w178] mode=indexing
          n138 = TDMS Get Properties(10:w178, 11:w181) -> (4:→"property values":variant[], 6:→"property names":string[])  [unwired: 4 in, 4 out]
        }
        n139 = global write "ESA_Data_Analysis_Global_VIs.vi" "group names"(w164) -> ()
        n140 = global read "SiPM_Tests_Global_Var.vi" "TDMS file array"() -> (w167:refnum<k34>[])
        n141 = Build Array (concatenate)(w167, w165) -> (w166:refnum<k34>[])
        n142 = global write "SiPM_Tests_Global_Var.vi" "TDMS file array"(w166) -> ()
      }
    }
    n143 = Or(x="Close Session", y=w12) -> (x .or. y?=w13:bool)
    n144 = local read "tdms file out"() -> (w14:refnum<k34>)
  }
  n145 = TDMS Close(11:w9) -> (0:w3:errorcluster)  [unwired: 1 in, 1 out]
  n146 = call <vilib>:"Simple Error Handler.vi"("type of dialog (OK msg:1)"=w2, "error in (no error)"=w3) -> ()  [unwired: 3 in, 5 out]
